vi "PagesLabelChange.vi"(8 "Array":string[](array[string]), 11 "Pages":refnum<vi>[](array[refnum])) -> ()   [LabVIEW 2015]
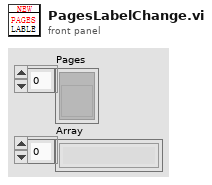
[diagram p1: front panel]
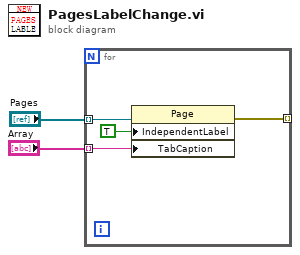
[diagram p0: block diagram]
diagram:
  n1 = for {
    tunnel: "Pages" -> [w6] mode=indexing
    tunnel: "Array" -> [w3] mode=indexing
    tunnel: [w4] -> _ mode=indexing
    n2 = property class="Page"(reference=w6, "IndependentLabel"=TRUE ("Page Visible"), "TabCaption"=w3) -> (error out=w4:errorcluster)  [unwired: 1 in, 1 out]
  }
